vi "Stop Background Loop.vi"(8 "error in (no error)":errorcluster, 11 "Worker Actor in":refnum<class "Worker Actor.lvclass">) -> (0 "error out":errorcluster, 3 "Worker Actor out":refnum<class "Worker Actor.lvclass">)   [LabVIEW 2021, in "Worker Actor.lvclass"]
uses:
  Worker Actor.lvclass
  NHMFL_Core/Libraries/Instruments/Instrument Driver/Worker State.ctl
  Worker Actor.lvclass/Worker Actor.ctl
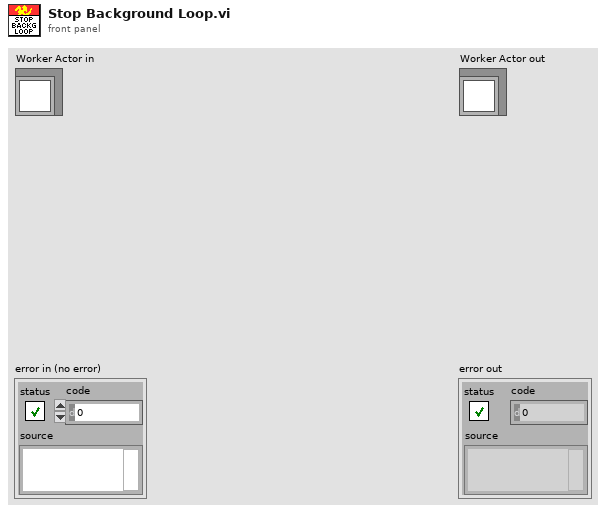
[diagram p1: front panel]
types:
  T1 = typedef "Worker State.ctl" = enum16{"Idle", "Starting", "Working", "Stopping"}
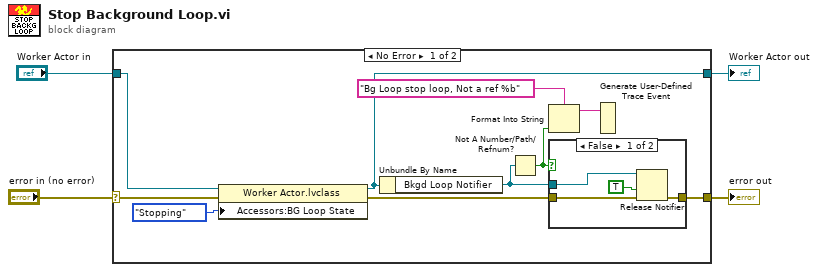
[diagram p0: block diagram]
diagram:
  n1 = case shown="No Error" "error in (no error)" {
    selector: "error in (no error)" -> [w13 w21]
    tunnel: [w12 w21] -> w3
    tunnel: [w6 w20] -> w1
    tunnel: "Worker Actor in" -> [w7 w20]
    frame No Error {
      n2 = property class="Worker Actor.lvclass"(reference=w7, error in=w13, "Accessors:BG Loop State"=Worker_State."Stopping" ("BG Loop State")) -> (reference out=w6:refnum<class "Worker Actor.lvclass">, error out=w8:errorcluster)
      n3 = Unbundle By Name(w6) -> ("Bkgd Loop Notifier"=w14:refnum<notifier>)
      n4 = Not A Number/Path/Refnum?(number/path/refnum=w14) -> (NaN/Path/Refnum?=w10:bool)
      n5 = Format Into String(format string="Bg Loop stop loop, Not a ref %b" ("trace string"), w10) -> (resulting string=w9:string)  [unwired: 2 in, 1 out]
      n6 = case shown="False" w10 {
        tunnel: w14 -> [w18 _]
        tunnel: w8 -> [w17 w19]
        tunnel: [w15 w19] -> w12
        frame False {
          n7 = Release Notifier(notifier=w18, force destroy? (F)=TRUE, error in (no error)=w17) -> (error out=w15:errorcluster)  [unwired: 2 out]
        }
        frame True {
        }
      }
      n8 = Generate User-Defined Trace Event(2:w9) -> ()  [unwired: 1 in]
    }
    frame Error {
    }
  }
  "error out" <- w3
  "Worker Actor out" <- w1
